vi "svx_Colormap Text Set.vi"(4 "BG color(transparent)":u32(colorbox)=16777216, 6 "text color(black)":u32(colorbox), 7 "text":string, 8 "Size":i16, 10 "origin":cluster{"x":i16, "y":i16}, 11 "picture":picture) -> (3 "new picture":picture)   [LabVIEW 2017, in "SVX Colormap.xctl"]
uses:
  <vilib>/addons/_XControls/Colormap/SVX Colormap.xctl
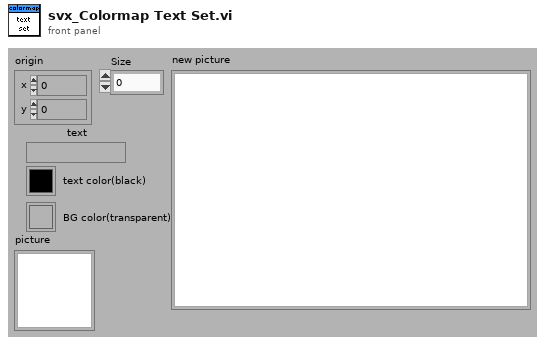
[diagram p1: front panel]
types:
  T1 = cluster{"Font Name:":string, "Size":i16, "Strikeout?":bool, "Italic?":bool, "Underline?":bool, "Outline?":bool, "Shadow?":bool, "Bold?":bool}
  T2 = enum16{"User-specified Font", "Application Font", "System Font", "Dialog Font"}
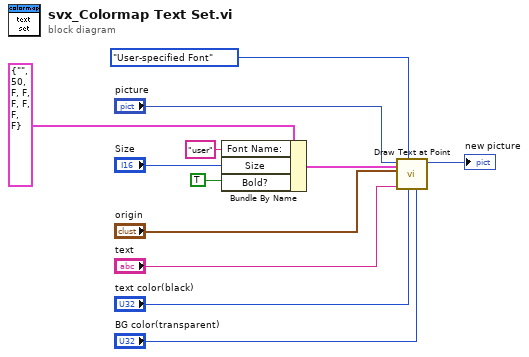
[diagram p0: block diagram]
diagram:
  n1 = Bundle By Name(cluster=T1 {"Font Name:"="", "Size"=50, "Strikeout?"=FALSE, "Italic?"=FALSE, "Underline?"=FALSE, "Outline?"=FALSE, "Shadow?"=FALSE, "Bold?"=FALSE} ("[user-specified font]"), "Font Name:"="user", "Size"="Size", "Bold?"=TRUE) -> (w9:T1)
  n2 = call <vilib>:"Draw Text at Point.vi"("BG color(transparent)"="BG color(transparent)", "[user-specified font]"=w9, "text color(black)"="text color(black)", "desired font(Application)"=T2."User-specified Font", "text"="text", "origin"="origin", "picture"="picture") -> ("new picture"=→"new picture":picture)  [unwired: 3 in, 1 out]
